vi "WS_PartNumberRef.vi"(1 "BCTYPE":i8, 2 "SerialNumber":string) -> (0 "AssemblyPartNumber":string)   [LabVIEW 2022 SP3]
uses:
  C:/Users/K90011729/OneDrive - Kimball Electronics/Desktop/Proyectos/IPB2 Test secuence/WsConnector/WSConnector.dll
  WSConnector.dll
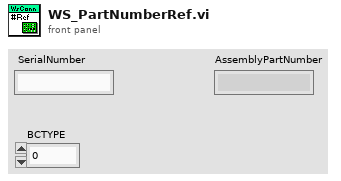
[diagram p1: front panel]
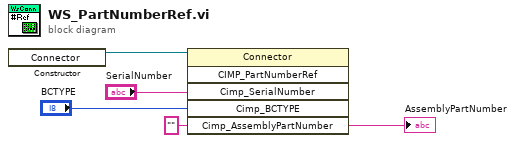
[diagram p0: block diagram]
diagram:
  n1 = constructor class="Connector"() -> (reference out=w5:refnum<k24>)  [unwired: 3 in, 2 out]
  n2 = invoke class="Connector" method="CIMP_PartNumberRef"(reference=w5, "Cimp_SerialNumber"="SerialNumber", "Cimp_BCTYPE"="BCTYPE", "Cimp_AssemblyPartNumber"="") -> ("Cimp_AssemblyPartNumber"=→"AssemblyPartNumber":string)  [unwired: 2 in, 5 out]
